vi "UDPtester_v1.vi"() -> ()   [LabVIEW 2016]
panel:
  in  "nums2send":dbl[](array[numeric])=[0.0, 0.0, 0.0, 0.0]
  out "double precision float":dbl[](array[numeric])
  in  "stop":bool
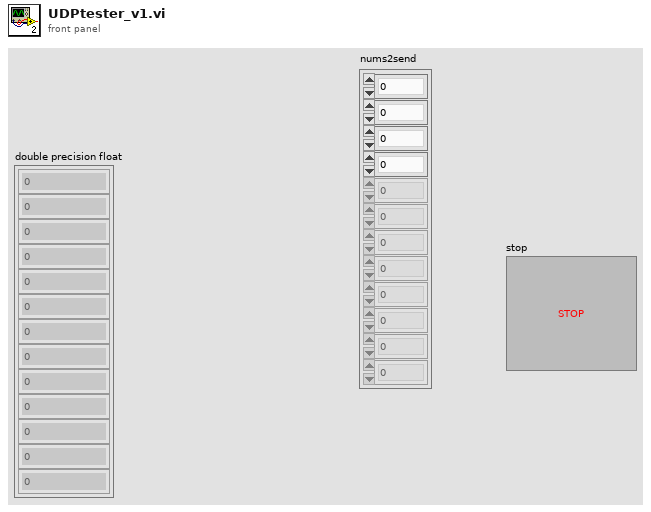
[diagram p1: front panel]
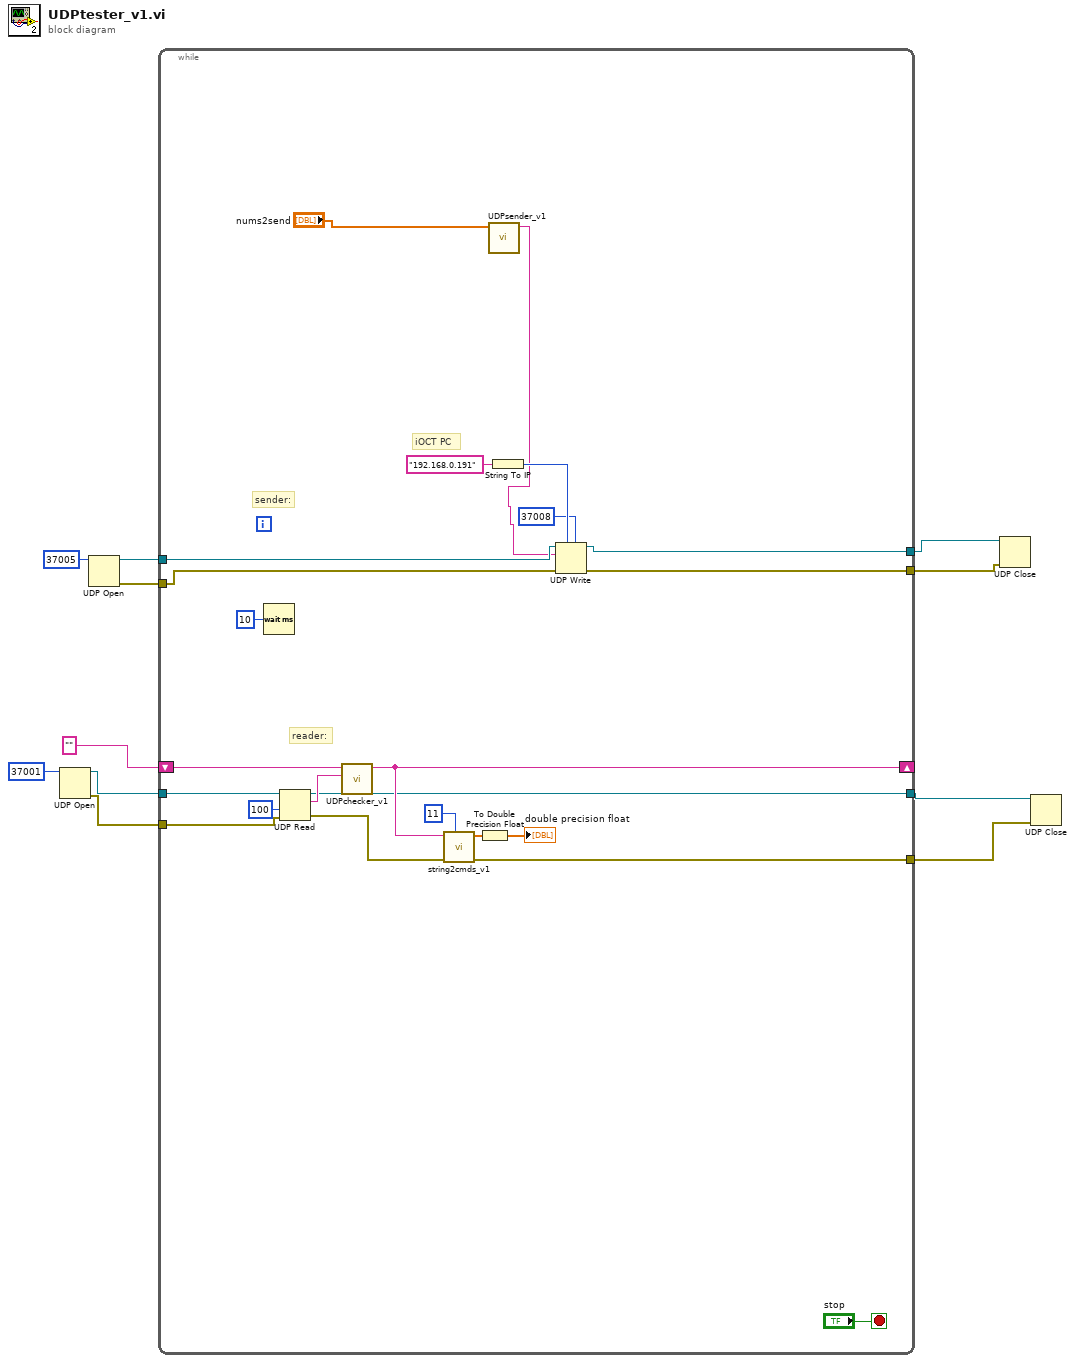
[diagram p0: block diagram]
diagram:
  n1 = UDP Open(11:u16 37001 ("port")) -> (port=w10:refnum<k16>, 0:w9:errorcluster)  [unwired: 4 in, 1 out]
  n2 = UDP Open(11:u16 37005 ("port")) -> (port=w5:refnum<k16>, 0:w4:errorcluster)  [unwired: 4 in, 1 out]
  n3 = while {
    tunnel: w10 -> [w27]
    tunnel: w9 -> [w26]
    shift-right: [w24] -> _
    shift-left: "" ("input string") -> [w25]
    tunnel: [w23] -> w7
    tunnel: [w22] -> w6
    tunnel: w5 -> [w21]
    tunnel: w4 -> [w20]
    tunnel: [w15] -> w2
    tunnel: [w14] -> w1
    stop <- "stop" stop-if-true
    # "iOCT PC"
    # "sender:"
    # "reader:"
    n4 = Wait (ms)(milliseconds to wait=u32 10) -> ()  [unwired: 1 out]
    n5 = UDP Read(connection ID=w27, timeout ms (25000)=100, 8:w26) -> (data out=w31:string, error out=w22:errorcluster, 3:w23:refnum<k16>)  [unwired: 1 in, 2 out]
    n6 = call "UDPchecker_v1.vi"("new string"=w31, "old string"=w25) -> ("output string"=w24:string)  [unwired: 9 in]
    n7 = call "string2cmds_v1.vi"("numCmds"=11, "input string"=w24) -> ("output cmds"=w30:sgl[])  [unwired: 9 in]
    n8 = To Double Precision Float(number=w30) -> (double precision float=→"double precision float":dbl[])
    n9 = call "UDPsender_v1.vi"("nums2send"="nums2send") -> ("string2send"=w12:string)  [unwired: 10 in]
    n10 = String To IP(1:"192.168.0.191" ("name")) -> (0:w17:u32)
    n11 = UDP Write(address=w17, port or service name=u16 37008, connection ID=w21, data in=w12, 8:w20) -> (error out=w14:errorcluster, 3:w15:refnum<k16>)  [unwired: 1 in]
  }
  n12 = UDP Close(connection ID=w2, 8:w1) -> ()  [unwired: 2 out]
  n13 = UDP Close(connection ID=w7, 8:w6) -> ()  [unwired: 2 out]
